vi "post.vi"(6 "request specific headers":T1[](array[typedef]), 7 "timeout (ms)":i32=10000, 8 "error in (no error)":errorcluster, 9 "request body":string, 10 "path":string, 11 "reqwest in":refnum<class "reqwest.lvclass">) -> (0 "error out":errorcluster, 2 "response":string, 3 "reqwest out":refnum<class "reqwest.lvclass">)   [LabVIEW 2020, in "reqwest.lvclass"]
uses:
  reqwest.lvclass
  reqwest.lvclass/reqwest.ctl
  shared-library/reqwest-labview.lvlib
  header.ctl
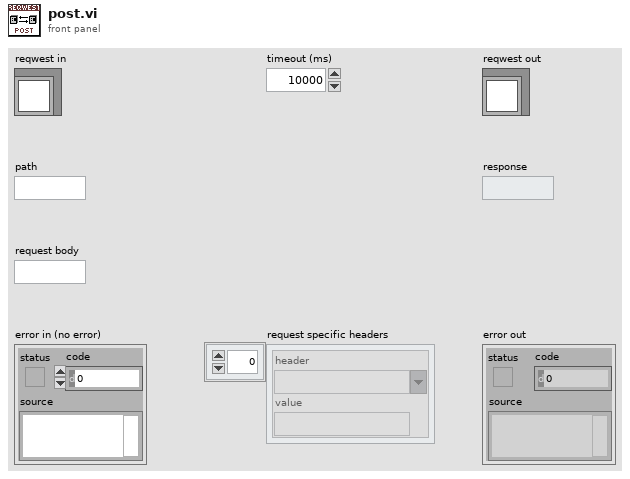
[diagram p1: front panel]
types:
  T1 = typedef "reqwest.lvclass/header.ctl" = cluster{"header":string, "value":string}
  T2 = typedef "reqwest.lvclass/private_data.ctl" = cluster{"Default Headers ([JSON])":T1[], "Base URL":string, "Authentication":cluster{"Username":string, "Password":string}}
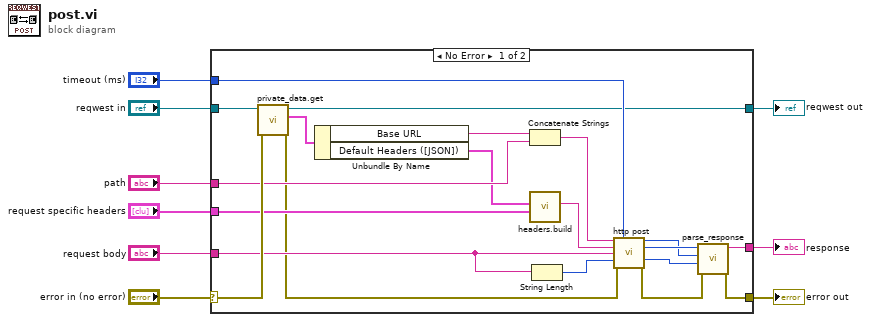
[diagram p0: block diagram]
diagram:
  n1 = case shown="No Error" "error in (no error)" {
    selector: "error in (no error)" -> [w28 w31]
    tunnel: [w11 w31] -> w8
    tunnel: [w16 w30] -> w6
    tunnel: "reqwest in" -> [w29 w30]
    tunnel: "path" -> [w25 _]
    tunnel: "request specific headers" -> [w23 _]
    tunnel: "request body" -> [w20 _]
    tunnel: "timeout (ms)" -> [w17 _]
    tunnel: [w10 _] -> w2
    frame No Error {
      n2 = call "private_data.get.vi"("error in (no error)"=w28, "reqwest in"=w29) -> ("error out"=w18:errorcluster, "private data"=w27:T2, "reqwest out"=w16:refnum<class "reqwest.lvclass">)  [unwired: 7 in]
      n3 = Unbundle By Name(w27) -> ("Base URL"=w26:string, "Default Headers ([JSON])"=w24:T1[])
      n4 = Concatenate Strings(w26, w25) -> (w22:string)
      n5 = call "headers.build.vi"("request specific headers"=w23, "default headers"=w24) -> ("Headers JSON"=w21:string)  [unwired: 9 in]
      n6 = String Length(string=w20) -> (length=w19:i32)
      n7 = call "http post.vi"("url"=w22, "timeout_ms"=w17, "headers_json"=w21, "body_ptr"=w20, "body_len"=w19, "error in (no error)"=w18) -> ("response_len_out"=w14:i32, "status_out"=w15:u32, "handle_out"=w13:u32, "error out"=w12:errorcluster)  [unwired: 5 in, 1 out]
      n8 = call "parse_response.vi"("error in"=w12, "handle_out"=w13, "response_len_out"=w14, "status_out"=w15) -> ("error out"=w11:errorcluster, "response"=w10:string)  [unwired: 6 in]
    }
    frame Error {
    }
  }
  "error out" <- w8
  "reqwest out" <- w6
  "response" <- w2
